vi "generate_DAC_voltages_V3.vi"(7 "focus mode?":bool, 8 "derived values":T1, 9 "scan specification":T4={"x amplitude"=0, "x resolution (pixels)"=0, "x offset fly-forward (iterations)"=0, "x offset fly-back (iterations)"=0, "y resolution (nr. of lines)"=0, "y step size"=0, "iterations per pixel"=0, "number of frames"=0, "y offset (pixels)"=0, "number of y-brake lines  (before y-fly-back)"=0, "number y-brake lines (after y-fly-back)"=0, "number of y-fly-back steps"=8, "lines per z step"=0, "number of z/intensity tuples"=0, "number of repetitions (volumes or planes)"=0, "z step size derived"=0, "choose the beginning of z scan"=FALSE, "number of frames (settings)"=0, "FPGA trajectory?"=FALSE}, 10 "counter cluster in":T2, 11 "resonant trigger":bool) -> (0 "acquire?":bool, 1 "fly-back acquisition phase?":bool, 2 "counter cluster out":T2, 3 "DAC voltages":T3 {"ch6" max=4095 step=1; "ch5" max=4095 step=1; "ch4" max=4095 step=1; "ch3" max=4095 step=1; "ch2" max=4095 step=1; "ch1" max=4095 step=1; "ch0" max=4095 step=1})   [LabVIEW 2010]
uses:
  scan_specification_cluster.ctl
  common_typedefs/DAC_voltage_cluster.ctl
  counter_cluster.ctl
  derived_values_cluster.ctl
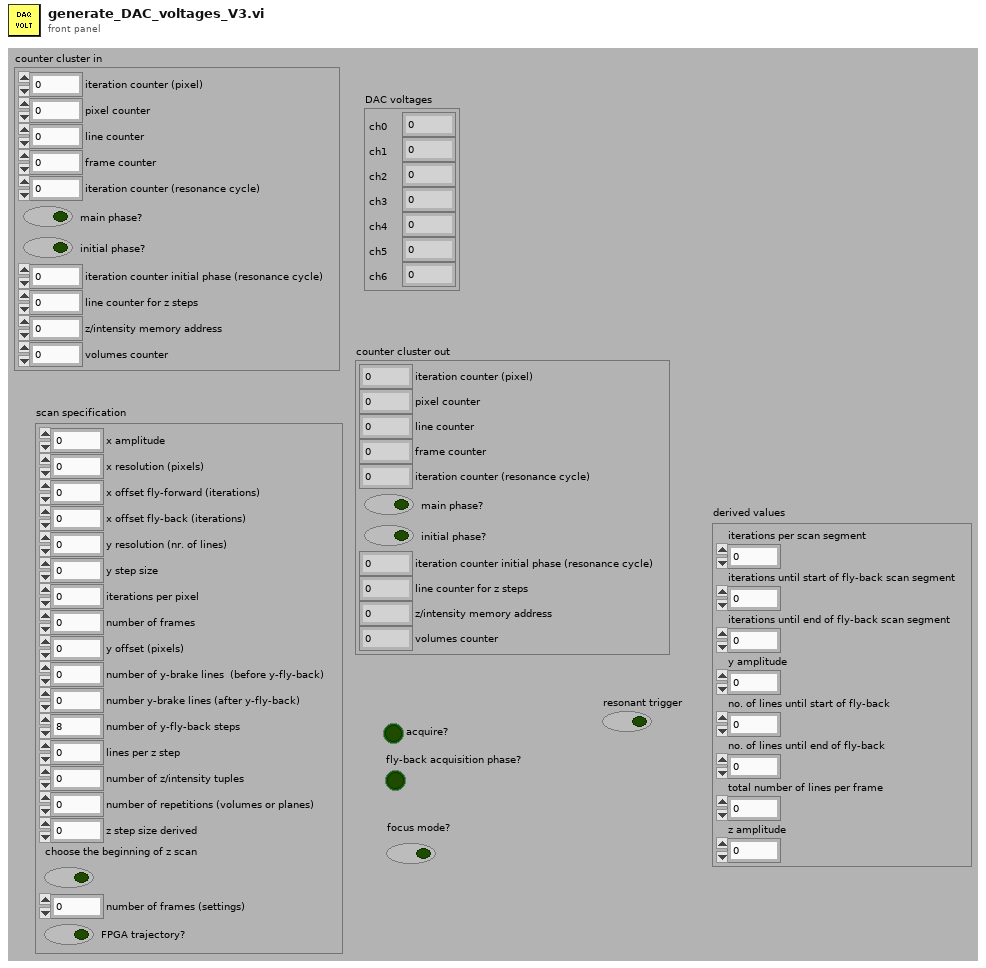
[diagram p1: front panel]
types:
  T1 = typedef "derived_values_cluster.ctl" = cluster{"iterations per scan segment":u16, "iterations until start of fly-back scan segment":u16, "iterations until end of fly-back scan segment":u16, "y amplitude":u16, "no. of lines until start of fly-back":u16, "no. of lines until end of fly-back":u16, "total number of lines per frame ":u16, "z amplitude":u16}
  T2 = typedef "counter_cluster.ctl" = cluster{"iteration counter (pixel)":u16, "pixel counter":u16, "line counter":u16, "frame counter":u16, "iteration counter (resonance cycle)":u16, "main phase?":bool, "initial phase?":bool, "iteration counter initial phase (resonance cycle)":u16, "line counter for z steps":u16, "z/intensity memory address":u32, "volumes counter":u16}
  T3 = typedef "DAC_voltage_cluster.ctl" = cluster{"ch0":u16, "ch1":i16, "ch2":i16, "ch3":u16, "ch4":u16, "ch5":u16, "ch6":u16}
  T4 = typedef "scan_specification_cluster.ctl" = cluster{"x amplitude":u16, "x resolution (pixels)":u16, "x offset fly-forward (iterations)":u16, "x offset fly-back (iterations)":u16, "y resolution (nr. of lines)":u16, "y step size":u16, "iterations per pixel":u16, "number of frames":i32, "y offset (pixels)":u16, "number of y-brake lines  (before y-fly-back)":u16, "number y-brake lines (after y-fly-back)":u16, "number of y-fly-back steps":u16, "lines per z step":u16, "number of z/intensity tuples":u16, "number of repetitions (volumes or planes)":i32, "z step size derived":u16, "choose the beginning of z scan":bool, "number of frames (settings)":i32, "FPGA trajectory?":bool}
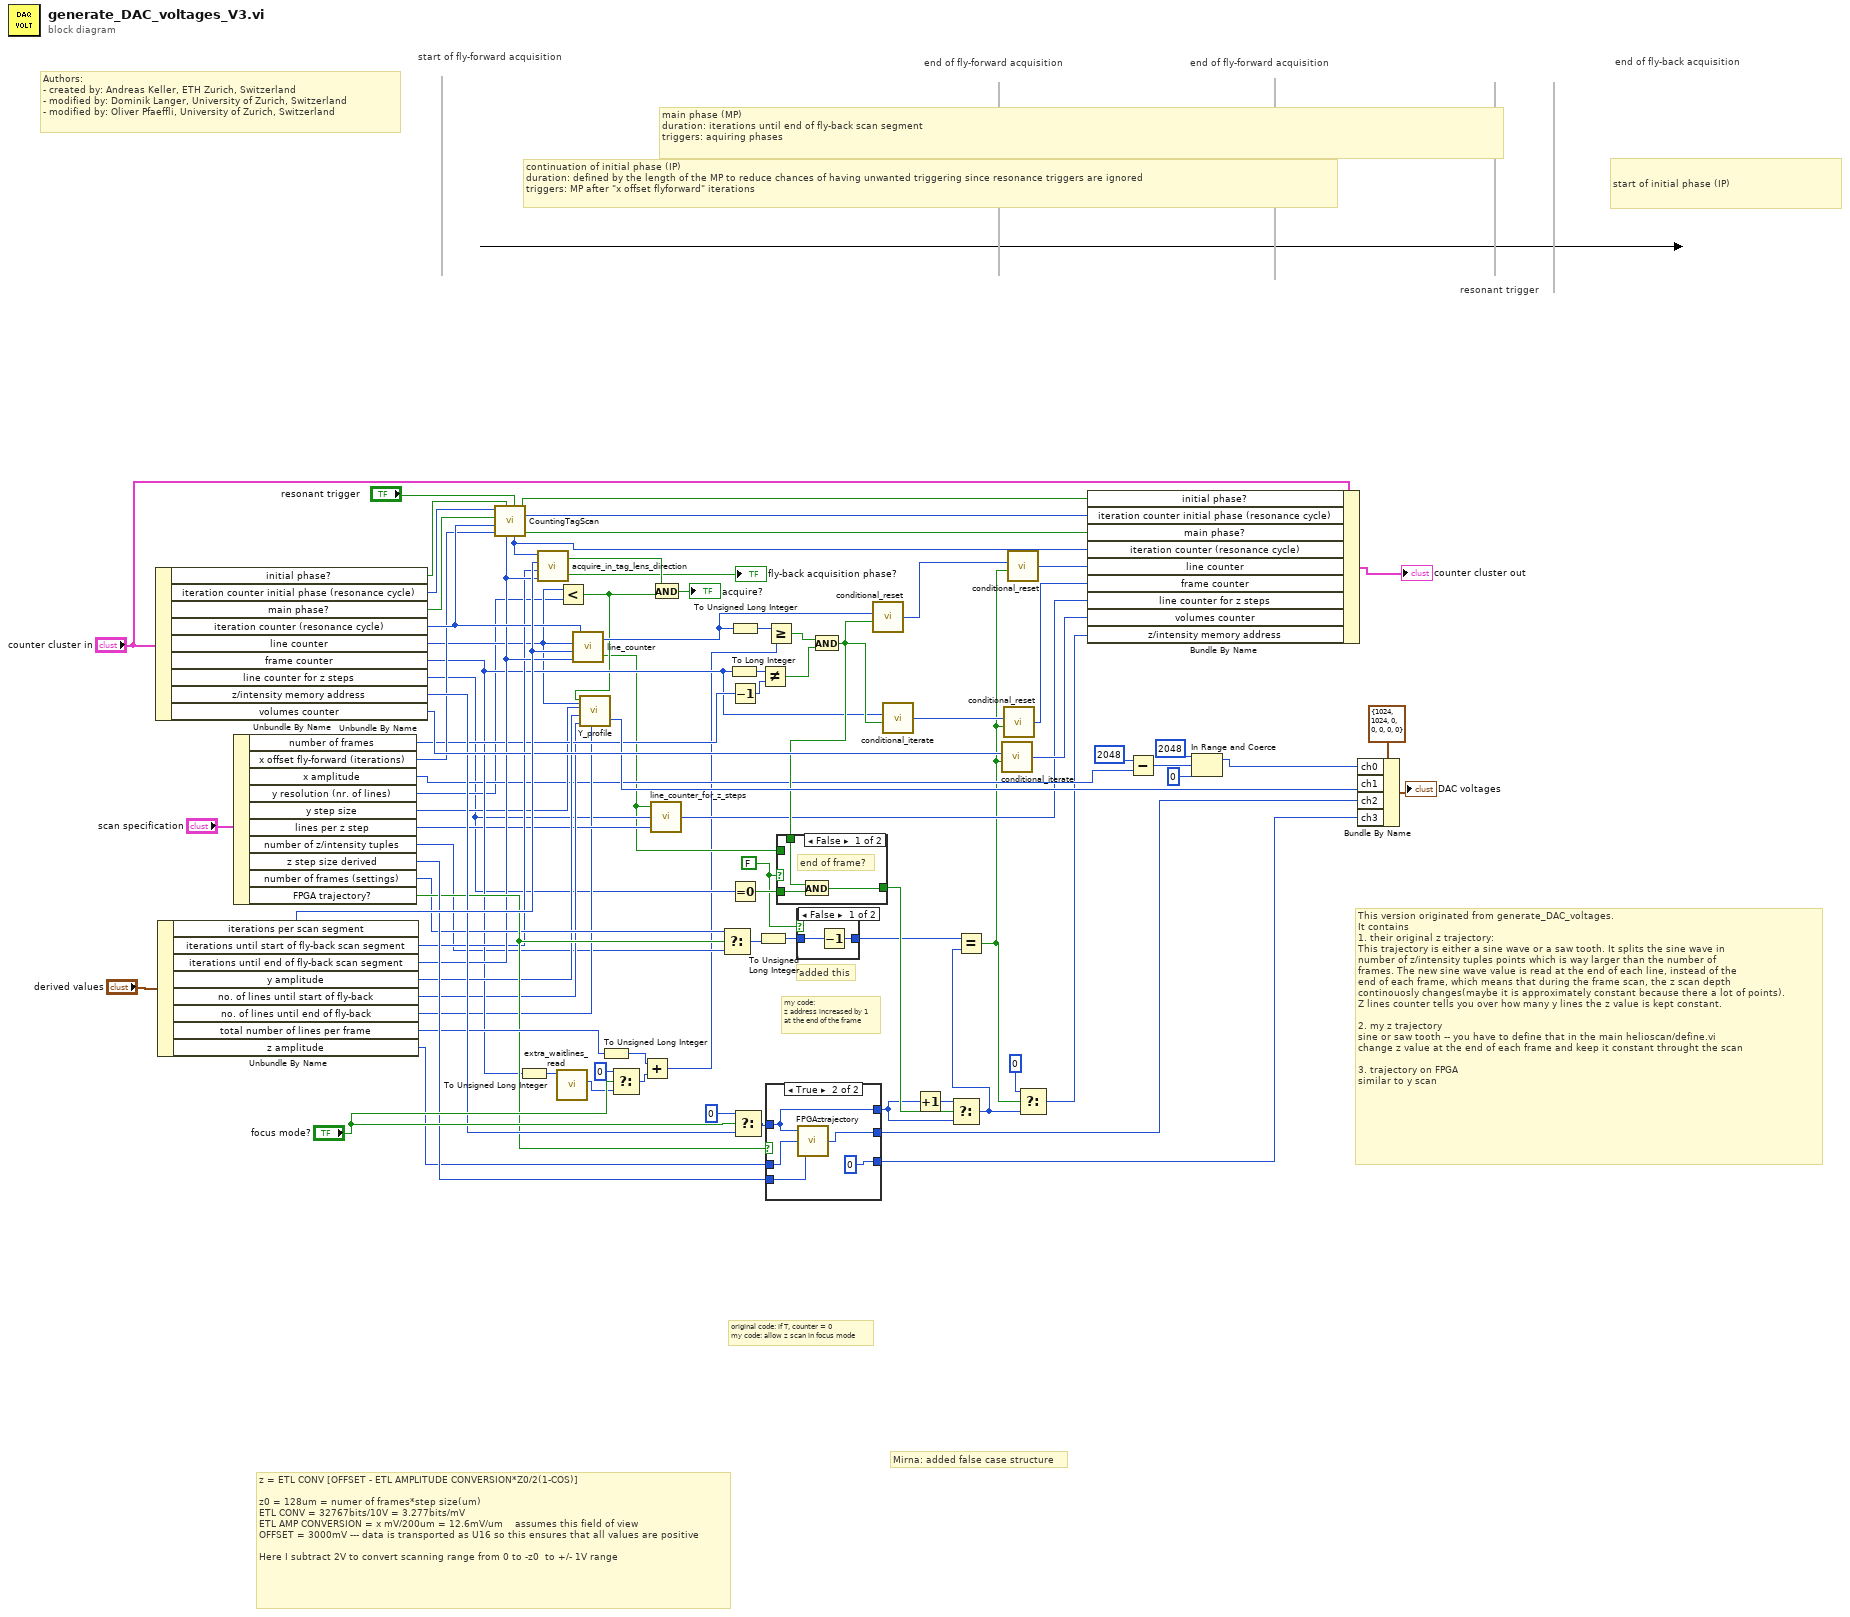
[diagram p0: block diagram]
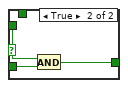
[diagram p3: hidden frame]
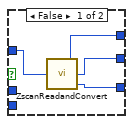
[diagram p4: hidden frame]
diagram:
  w40 = FALSE
  # "This version originated from generate_DAC_voltages.\nIt contains \n1. their original z trajectory:\nThis trajectory is either a sine wave or a saw tooth. It splits the sine wave in\nnumber of z/intensity tuples points which is way larger than the number of\nframes. The new sine wave value is read at the end of each line, instead of the\nend of each frame, which means that during the frame scan, the z scan depth \ncontinouosly changes(maybe it is approximately constant because there a lot of points).\nZ lines counter tells you over how many y lines the z value is kept constant.\n\n2. my z trajectory\nsine or saw tooth -- you have to define that in the main helioscan/define.vi\nchange z value at the end of each frame and keep it constant throught the scan\n\n3. trajectory on FPGA\nsimilar to y scan"
  # "added this"
  # "z = ETL CONV [OFFSET - ETL AMPLITUDE CONVERSION*Z0/2(1-COS)]\n\nz0 = 128um = numer of frames*step size(um)\nETL CONV = 32767bits/10V = 3.277bits/mV\nETL AMP CONVERSION = x mV/200um = 12.6mV/um    assumes this field of view\nOFFSET = 3000mV --- data is transported as U16 so this ensures that all values are positive\n\nHere I subtract 2V to convert scanning range from 0 to -z0  to +/- 1V range"
  # "my code:\nz address increased by 1\nat the end of the frame"
  # "original code: if T, counter = 0\nmy code: allow z scan in focus mode"
  # "Mirna: added false case structure"
  # "start of initial phase (IP)"
  # "continuation of initial phase (IP)\nduration: defined by the length of the MP to reduce chances of having unwanted triggering since resonance triggers are ignored\ntriggers: MP after \"x offset flyforward\" iterations"
  # "end of fly-back acquisition"
  # "end of fly-forward acquisition"
  # "end of fly-forward acquisition"
  # "start of fly-forward acquisition"
  # "main phase (MP)\nduration: iterations until end of fly-back scan segment\ntriggers: aquiring phases"
  # "resonant trigger"
  # "Authors: \n- created by: Andreas Keller, ETH Zurich, Switzerland\n- modified by: Dominik Langer, University of Zurich, Switzerland\n- modified by: Oliver Pfaeffli, University of Zurich, Switzerland"
  n1 = Unbundle By Name("counter cluster in") -> ("initial phase?"=w74:bool, "iteration counter initial phase (resonance cycle)"=w33:u16, "main phase?"=w59:bool, "iteration counter (resonance cycle)"=w32:u16, "line counter"=w23:u16, "frame counter"=w24:u16, "line counter for z steps"=w8:u16, "z/intensity memory address"=w54:u32, "volumes counter"=w61:u16)
  n2 = Unbundle By Name("derived values") -> ("iterations per scan segment"=w73:u16, "iterations until start of fly-back scan segment"=w30:u16, "iterations until end of fly-back scan segment"=w31:u16, "y amplitude"=w37:u16, "no. of lines until start of fly-back"=w21:u16, "no. of lines until end of fly-back"=w19:u16, "total number of lines per frame"=w48:u16, "z amplitude"=w38:u16)
  n3 = Unbundle By Name("scan specification") -> ("number of frames"=w25:i32, "x offset fly-forward (iterations)"=w28:u16, "x amplitude"=w17:u16, "y resolution (nr. of lines)"=w11:u16, "y step size"=w22:u16, "lines per z step"=w20:u16, "number of z/intensity tuples"=w13:u16, "z step size derived"=w49:u16, "number of frames (settings)"=w44:i32, "FPGA trajectory?"=w45:bool)
  n4 = call "CountingTagScan.vi"("resonant trigger"="resonant trigger", "initial phase?"=w74, "iteration counter initial phase (resonance cycle)"=w33, "main phase?"=w59, "iterations until end of fly-back scan segment"=w31, "iteration counter (resonance cycle)"=w32, "x offset fly-forward (iterations)"=w28) -> ("initial phase? OUT"=w35:bool, "iteration counter initial phase (resonance cycle) out"=w34:u16, "main phase? OUT"=w27:bool, "iteration counter (resonance cycle) out"=w2:u16)
  n5 = To Unsigned Long Integer(number=w24) -> (unsigned 32bit integer=w14:u32)
  n6 = call "acquire_in_tag_lens_direction.vi"("iterations until end of fly-back scan segment"=w31, "iterations until start of fly-back scan segment"=w30, "iterations per scan segment"=w73, "iteration counter (resonance cycle) out"=w2) -> ("flyback phase?"=→"fly-back acquisition phase?":bool, "acquire during flyforward or flyback phase?"=w76:bool)
  n7 = call "extra_waitlines_read.vi"("address extra waitlines IN"=w14) -> ("extra waitline data"=w42:u32)  [unwired: 9 in, 1 out]
  n8 = Less?(x=w23, y=w11) -> (x < y?=w9:bool)
  n9 = call "line_counter.vi"("iterations until end of fly-back scan segment"=w31, "iterations per scan segment"=w73, "line counter in"=w23, "iteration counter (resonance cycle)"=w32) -> ("end of line?"=w7:bool, "line counter out"=w12:u16)
  n10 = call "Y_profile.vi"("no. of lines until end of fly-back"=w19, "line counter"=w23, "no. of lines until start of fly-back"=w21, "y amplitude"=w37, "y step size"=w22, "true when line counter smaller than y resolution"=w9) -> ("y signal"=w58:i16)  [unwired: 1 in]
  n11 = To Unsigned Long Integer(number=w48) -> (unsigned 32bit integer=w46:u32)
  n12 = Select(t=u32 0, s="focus mode?", f=w42) -> (s? t:f=w63:u32)
  n13 = Add(x=w46, y=w63) -> (x+y=w6:u32)
  n14 = call "line_counter_for_z_steps.vi"("lines per z step"=w20, "line counter for z steps"=w8, "end of line?"=w7) -> ("line counter for z steps out"=w15:u16)
  n15 = And(x=w76, y=w9) -> (x .and. y?=→"acquire?":bool)
  n16 = Select(t=w44, s=w45, f=w13) -> (s? t:f=w53:i32)
  n17 = To Long Integer(number=w24) -> (32bit integer=w64:i32)
  n18 = To Unsigned Long Integer(number=w12) -> (unsigned 32bit integer=w43:u32)
  n19 = Decrement(x=w25) -> (x-1=w65:i32)
  n20 = Equal To 0?(x=w8) -> (x = 0?=w70:bool)
  n21 = Select(t=u32 0, s="focus mode?", f=w54) -> (s? t:f=w55:u32)
  n22 = To Unsigned Long Integer(number=w53) -> (unsigned 32bit integer=w71:u32)
  n23 = Not Equal?(x=w64, y=w65) -> (x != y?=w18:bool)
  n24 = Greater Or Equal?(x=w43, y=w6) -> (x >= y?=w66:bool)
  n25 = case shown="True" w45 {
    tunnel: [w87 u16 0 ("intensity")] -> w57
    tunnel: [w89 w90] -> w4
    tunnel: [w86 w93] -> w56
    tunnel: w55 -> [w88 w90]
    tunnel: w49 -> [_ w94]
    tunnel: w38 -> [_ w92]
    frame False {
      n26 = call "ZscanReadandConvert.vi"("z/intensity memory address"=w88) -> ("intensity profile"=w87:u16, "z profile"=w86:u16, "address out"=w89:u32)
    }
    frame True {
      n27 = call "FPGAztrajectory.vi"("z step size derived"=w94, "z amplitude"=w92, "z/intensity memory address"=w90) -> ("Z trajectory"=w93:i16)
    }
  }
  n28 = case shown="False" w40 {
    tunnel: w71 -> [w96 w97]
    tunnel: [w95 w97] -> w41
    frame False {
      n29 = Decrement(x=w96) -> (x-1=w95:u32)
    }
    frame True {
    }
  }
  n30 = And(x=w66, y=w18) -> (x .and. y?=w50:bool)
  n31 = case shown="False" w40 {
    tunnel: w70 -> [w100 w103]
    tunnel: w7 -> [_ w102]
    tunnel: [w99 w101] -> w47
    tunnel: w50 -> [w98 _]
    frame False {
      # "end of frame?"
      n32 = And(x=w98, y=w100) -> (x .and. y?=w99:bool)
    }
    frame True {
      n33 = And(x=w102, y=w103) -> (x .and. y?=w101:bool)
    }
  }
  n34 = call "conditional_reset.vi"("reset?"=w50, "number in"=w12) -> ("number out"=w68:u16)  [unwired: 4 in]
  n35 = call "conditional_iterate.vi"("iterate?"=w50, "number in"=w24) -> ("number out"=w51:u16)  [unwired: 4 in]
  n36 = Increment(x=w4) -> (x+1=w72:u32)
  n37 = Select(t=w72, s=w47, f=w4) -> (s? t:f=w3:u32)
  n38 = Equal?(x=w41, y=w3) -> (x = y?=w1:bool)
  n39 = call "conditional_iterate.vi"("iterate?"=w1, "number in"=w61) -> ("number out"=w69:u16)  [unwired: 4 in]
  n40 = call "conditional_reset.vi"("reset?"=w1, "number in"=w51) -> ("number out"=w52:u16)  [unwired: 4 in]
  n41 = call "conditional_reset.vi"("reset?"=w1, "number in"=w68) -> ("number out"=w67:u16)  [unwired: 4 in]
  n42 = Select(t=u32 0, s=w1, f=w3) -> (s? t:f=w5:u32)
  n43 = Bundle By Name(cluster="counter cluster in", "initial phase?"=w35, "iteration counter initial phase (resonance cycle)"=w34, "main phase?"=w27, "iteration counter (resonance cycle)"=w2, "line counter"=w67, "frame counter"=w52, "line counter for z steps"=w15, "volumes counter"=w69, "z/intensity memory address"=w5) -> (→"counter cluster out":T2)
  n44 = Subtract(x=u16 2048, y=w17) -> (x-y=w80:u16)
  n45 = In Range and Coerce(upper limit=u16 2048, x=w80, lower limit=u16 0) -> (coerced(x)=w79:u16)  [unwired: 1 out]
  n46 = Bundle By Name(cluster=T3 {"ch0"=1024, "ch1"=1024, "ch2"=0, "ch3"=0, "ch4"=0, "ch5"=0, "ch6"=0} ("DAC voltage"), "ch0"=w79, "ch1"=w58, "ch2"=w56, "ch3"=w57) -> (→"DAC voltages":T3)
